vi "Moving_Average.vi"(0 "Moving_Average":i32, 11 "Error_In":errorcluster) -> (4 "Moving_Average_Value":dbl, 15 "Error_Out":errorcluster)   [LabVIEW 2021]
doc: "This VI calculate Moving average from the generated data."
uses:
  Controls/Operation_Select_Stack.ctl
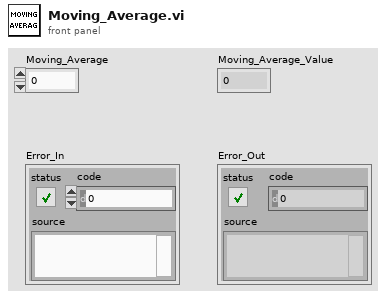
[diagram p1: front panel]
types:
  T1 = typedef "Operation_Select_Stack.ctl" = enum16{"Initialize", "Push", "Pop", "Preview"}
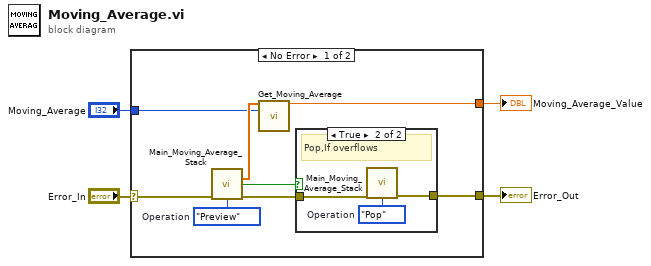
[diagram p0: block diagram]
diagram:
  n1 = case shown="No Error" "Error_In" {
    selector: "Error_In" -> [w12 w17]
    tunnel: [w9 w17] -> w3
    tunnel: "Moving_Average" -> [w7 _]
    tunnel: [w6 _] -> w1
    frame No Error {
      w5 = Operation_Select_Stack."Preview"  # Operation
      n2 = call "Main_Moving_Average_Stack.vi"("Error_In"=w12, "Operation"=w5) -> ("Generated_Data_Preview"=w8:dbl[], "Overflow"=w11:bool, "Error_Out"=w10:errorcluster)  [unwired: 9 in, 2 out]
      n3 = call "Get_Moving_Average.vi"("Generated_Data_Preview"=w8, "Moving_Average"=w7) -> ("Numeric"=w6:dbl)  [unwired: 13 in]
      n4 = case shown="True" w11 {
        tunnel: w10 -> [w13 w16]
        tunnel: [w13 w15] -> w9
        frame False {
        }
        frame True {
          w14 = Operation_Select_Stack."Pop"  # Operation
          # "Pop,If overflows"
          n5 = call "Main_Moving_Average_Stack.vi"("Error_In"=w16, "Operation"=w14) -> ("Error_Out"=w15:errorcluster)  [unwired: 9 in, 4 out]
        }
      }
    }
    frame Error {
    }
  }
  "Error_Out" <- w3
  "Moving_Average_Value" <- w1
